vi "Main - Root Path (FGV).vi"(6 "Action":T1=enum."Write", 8 "error in":errorcluster, 11 "Path in":path) -> (0 "error out":errorcluster, 3 "Path out":path)   [LabVIEW 2019]
uses:
  Controls/FGV States.ctl
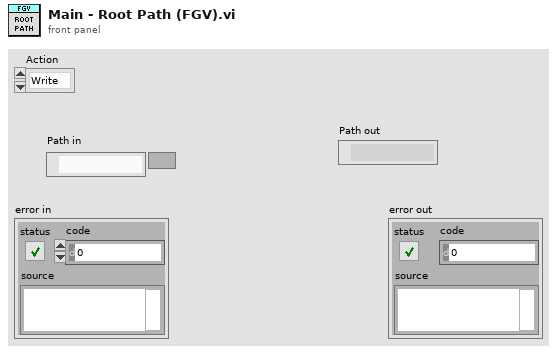
[diagram p1: front panel]
types:
  T1 = typedef "FGV States.ctl" = enum16{"Read", "Write"}
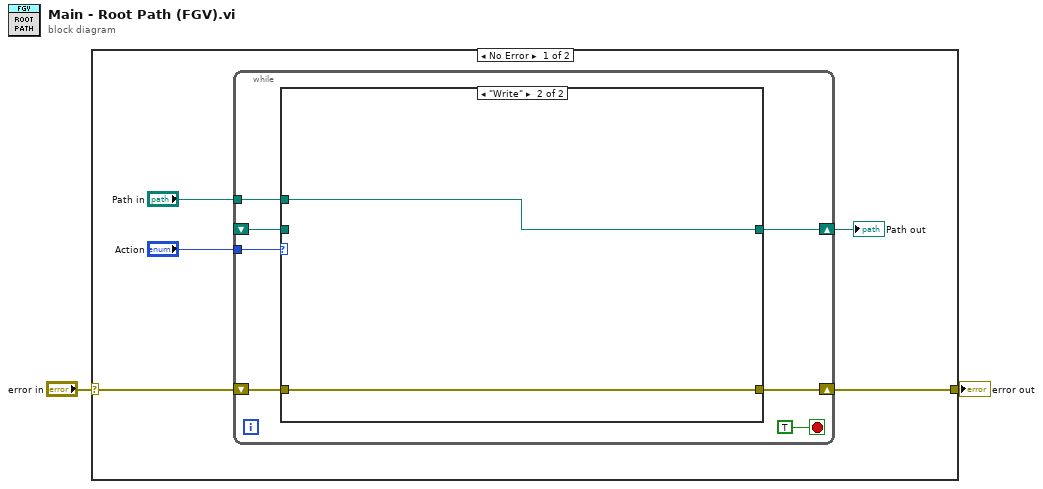
[diagram p0: block diagram]
diagram:
  n1 = case shown="No Error" "error in" {
    selector: "error in" -> [w7 w19]
    tunnel: [w6 w19] -> w1
    frame No Error {
      n2 = while {
        tunnel: "Action" -> [w12]
        shift-right: [w13] -> w6
        shift-left: w7 -> [w14]
        tunnel: "Path in" -> [w11]
        shift-right: [w10] -> w3
        shift-left: _ -> [w9]
        stop <- TRUE stop-if-true
        n3 = case shown="\"Write\"" w12 {
          tunnel: w14 -> [w16 w17]
          tunnel: [w16 w17] -> w13
          tunnel: w11 -> [_ w18]
          tunnel: [w15 w18] -> w10
          tunnel: w9 -> [w15 _]
          frame "Read", Default {
          }
          frame "Write" {
          }
        }
      }
      "Path out" <- w3
    }
    frame Error {
    }
  }
  "error out" <- w1
